vi "Classic Monitor.vi"(8 "error in (no error)":errorcluster, 10 "Enable Orphan Detection?":bool=TRUE) -> (0 "error out":errorcluster, 3 "Classic Monitor out":refnum<class "Classic Monitor.lvclass">)   [LabVIEW 2023, in "Monitored Actor.lvlib" / "Classic Monitor.lvclass"]
doc: "Configures the Classic AF monitor window.\n\nCopyright: MGI 2016\nAuthor: Derek Trepanier"
uses:
  Classic Monitor.lvclass
  Classic Monitor.lvclass/Classic Monitor.ctl
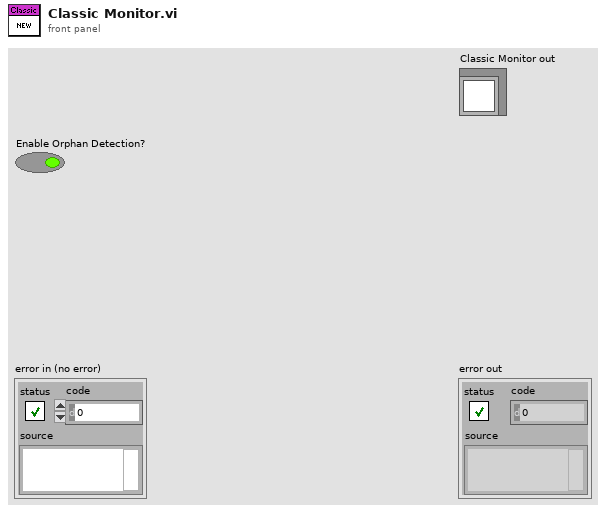
[diagram p1: front panel]
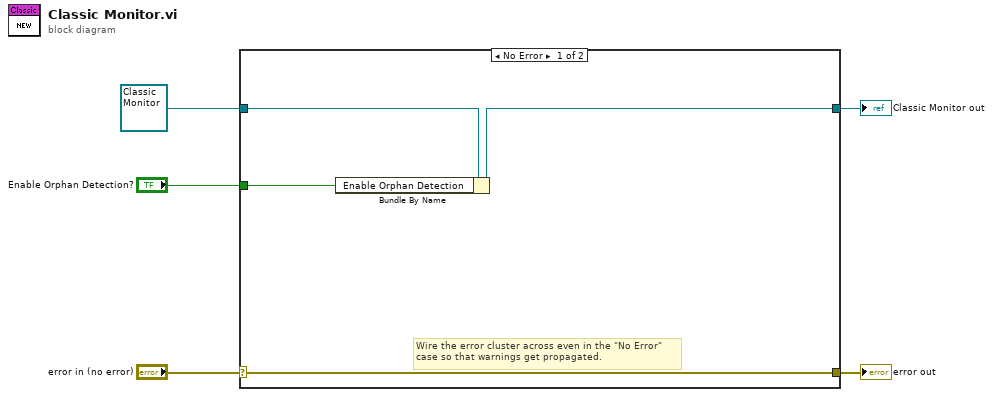
[diagram p0: block diagram]
diagram:
  n1 = case shown="No Error" "error in (no error)" {
    selector: "error in (no error)" -> [w8 w11]
    tunnel: [w8 w11] -> w4
    tunnel: [w7 w10] -> w2
    tunnel: refnum<class "Classic Monitor.lvclass"> refnum ("Classic Monitor in") -> [w9 w10]
    tunnel: "Enable Orphan Detection?" -> [w6 _]
    frame No Error {
      # "Wire the error cluster across even in the \"No Error\"\ncase so that warnings get propagated."
      n2 = Bundle By Name(cluster=w9, "Enable Orphan Detection"=w6) -> (w7:refnum<class "Classic Monitor.lvclass">)
    }
    frame Error {
    }
  }
  "error out" <- w4
  "Classic Monitor out" <- w2
